vi "TEST-SERIALIZE.vi"() -> ()   [LabVIEW 2019]
uses:
  Response--Variant--Cluster.ctl
  Response--String--Cluster.ctl
  83b9611c-e125-4a79-a28c-7d3b3a1c2440.vi
  eb13c5f8-5704-4e01-b19a-e5499a693321.vi
  35bd3d0d-1b36-4666-bfef-67306258898e.vi
  db572bd4-01e3-4c34-87d8-1273e3f61b28.vi
  9ae522ea-7a25-4ffe-8949-55076a4dedc3.vi
  1886c53c-c316-4cc4-aec7-e01830886c52.vi
  2ae47432-6b04-43af-b607-7b3945031cca.vi
  7945c8ed-bd74-4a6a-aaee-7dd52200f6b1.vi
  83b9611c-e125-4a79-a28c-7d3b3a1c2440.vi/16d22996-583c-4114-be7f-826d89ca4985.vi
  9ae522ea-7a25-4ffe-8949-55076a4dedc3.vi/34417eb6-c264-4261-ab76-2576b9b9ebac.vi
  lv-venv/lv.lib/vi.lib/JDP Science/JSONtext/Variant to JSON Text.vi
  <vilib>/Utility/sysdir.llb/Get System Directory.vi
  lv-venv/lv.lib/vi.lib/JDP Science/JSONtext/JSON text to Variant.vi
  lv-venv/lv.lib/vi.lib/JDP Science/JSONtext/LVClass Serializer/JSONtext LVClass Serializer.lvclass
  lv-venv/lv.lib/vi.lib/addons/_JKI.lib/Serialization/JSON/JKI JSON Serialization.lvlib
panel:
  out "serialize":dbl
  out "Numeric":i32
  out "spreadsheet string":string
  out "XY Graph":cluster{i32[], dbl[]}[](graph)
  out "Array":i32[](array[numeric])
  out "data":i32[](array[numeric])
  out "serialize JSON":dbl[](array[numeric]) format="%#_6p"
  out "{JSON}":string
  out "id":string
  out "parse JSON":dbl[](array[numeric]) format="%#_6p"
  in  "Enum":T1(ring)
  out "x = y?":bool
  in  "Max Array Size":i32=100 format="%.0p"
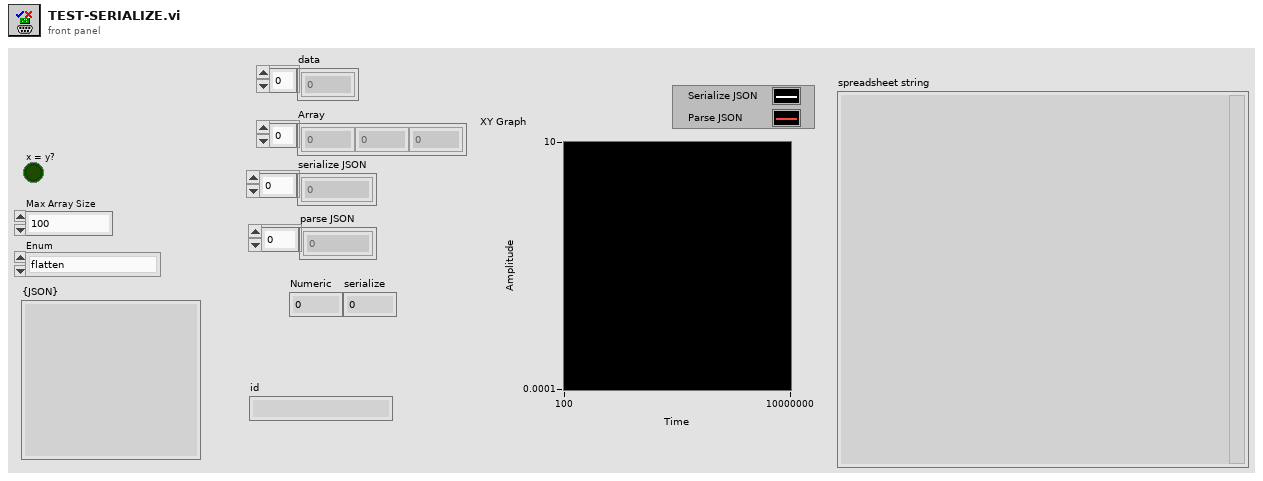
[diagram p1: front panel]
types:
  T1 = enum16{"flatten", "JKI JSON", "JKI JSON + flatten", "JSONtext", "JSONtext + flatten", "myJSON + flatten", "PythonModule"}
  T2 = typedef "Response--Variant--Cluster.ctl" = cluster{"jsonrpc":string, "result":variant, "id":string}
  T3 = typedef "Response--String--Cluster.ctl" = cluster{"jsonrpc":string, "result":string, "id":string}
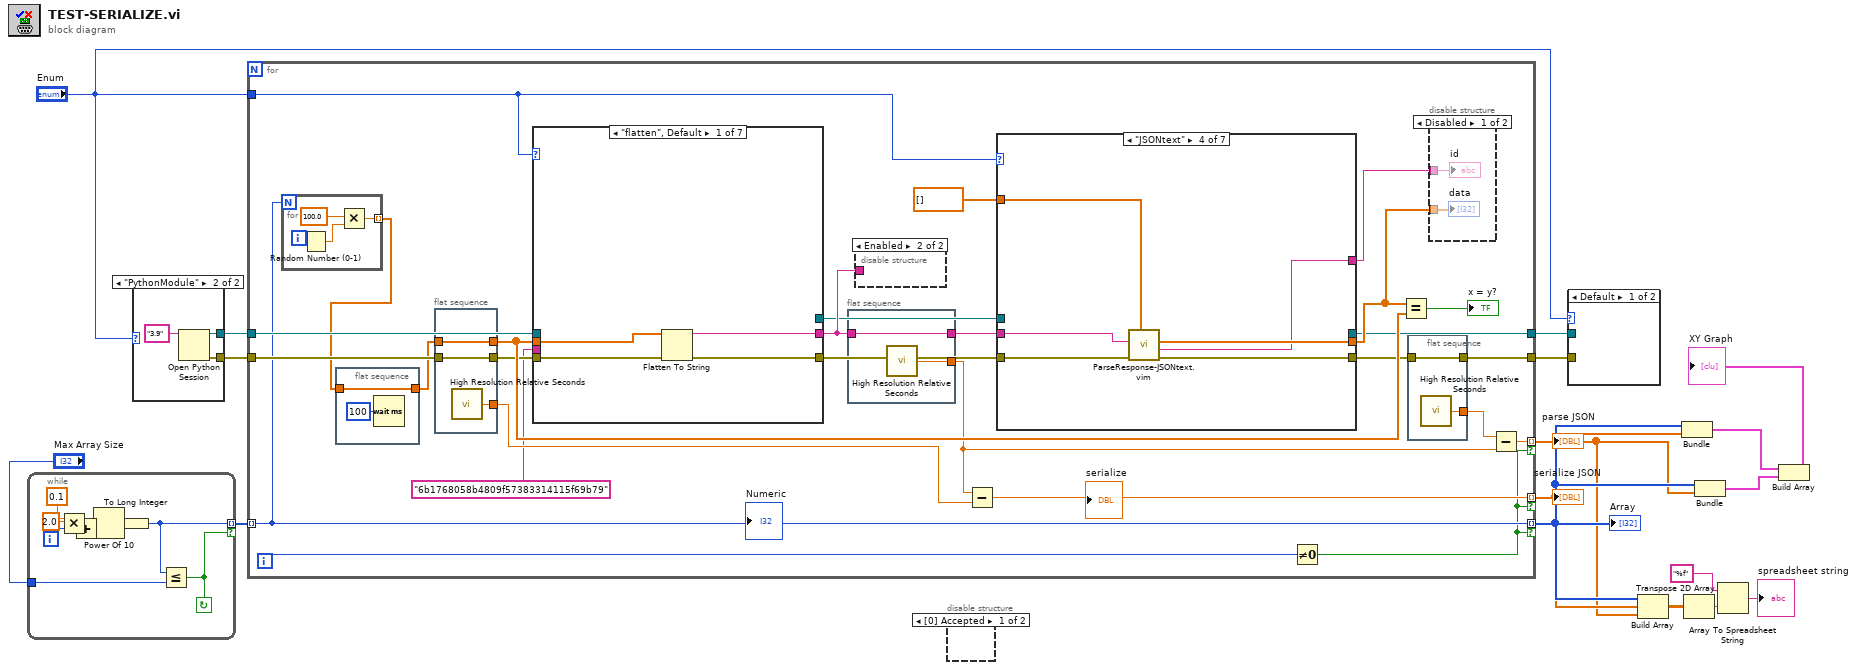
[diagram p0: block diagram]
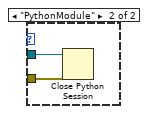
[diagram p3: hidden frame]
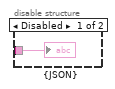
[diagram p5: hidden frame]
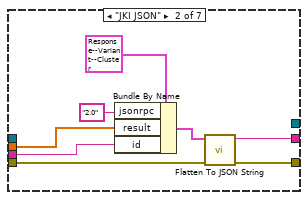
[diagram p6: hidden frame]
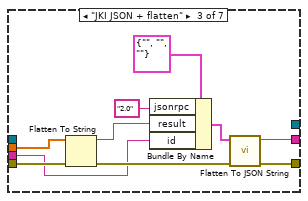
[diagram p7: hidden frame]
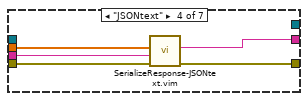
[diagram p8: hidden frame]
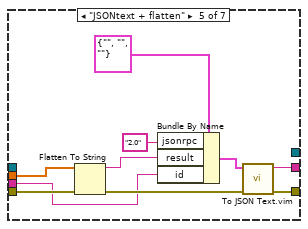
[diagram p9: hidden frame]
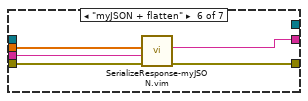
[diagram p10: hidden frame]
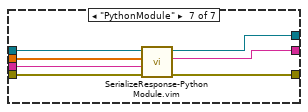
[diagram p11: hidden frame]
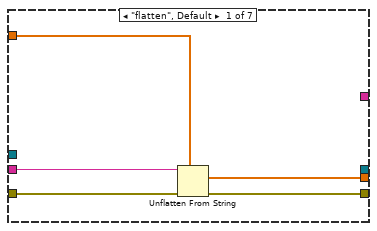
[diagram p12: hidden frame]
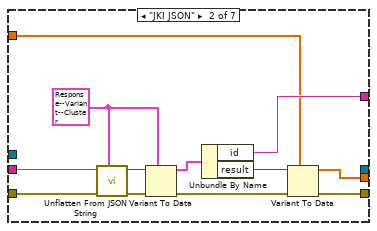
[diagram p13: hidden frame]
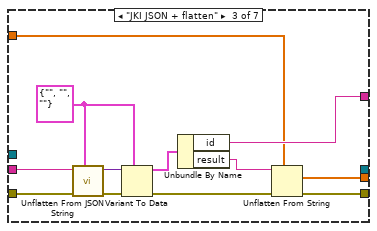
[diagram p14: hidden frame]
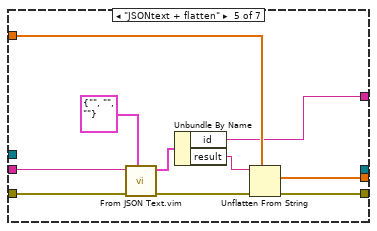
[diagram p15: hidden frame]
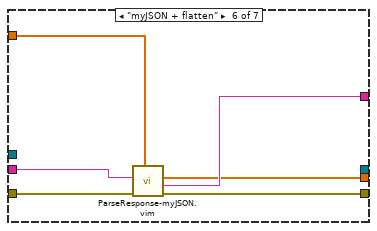
[diagram p16: hidden frame]
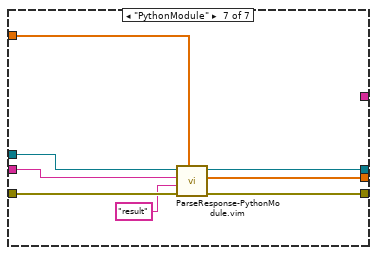
[diagram p17: hidden frame]
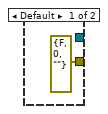
[diagram p18: hidden frame]
diagram:
  n1 = while {
    tunnel: [w18] -> w14 mode=indexing if=w23
    tunnel: "Max Array Size" -> [w22]
    i -> [w26]
    stop <- w23 continue-if-true
    n2 = Multiply(x=0.1, y=w26) -> (x*y=w24:dbl)
    n3 = Add(x=w24, y=2.0) -> (x+y=w20:dbl)
    n4 = Power Of 10(x=w20) -> (10^x=w21:dbl)
    n5 = To Long Integer(number=w21) -> (32bit integer=w18:i32)
    n6 = Less Or Equal?(x=w18, y=w22) -> (x <= y?=w23:bool)
  }
  n7 = case shown="\"PythonModule\"" "Enum" {
    tunnel: [errorcluster {"status"=FALSE, "code"=0, "source"=""} ("error in (no error)") w29] -> w17
    tunnel: [_ w28] -> w16
    frame Default {
    }
    frame "PythonModule" {
      n8 = Open Python Session(python version="3.9" ("Python version")) -> (session out=w28:refnum<k35>, error out=w29:errorcluster)  [unwired: 2 in]
    }
  }
  n9 = for {
    tunnel: [w49] -> w6 mode=indexing if=w35
    tunnel: [w45] -> w5 mode=indexing if=w35
    tunnel: w17 -> [w42]
    tunnel: w16 -> [w41]
    tunnel: "Enum" -> [w40]
    tunnel: w14 -> [w37] mode=indexing
    tunnel: [w37] -> w7 mode=indexing if=w35
    tunnel: [w34] -> w10
    tunnel: [w33] -> w9
    i -> [w36]
    n10 = for {
      N: w37 -> [_]
      tunnel: [w179] -> w31 mode=indexing
      n11 = Random Number (0-1)() -> (number: 0 to 1=w178:dbl)
      n12 = Multiply(x=100.0, y=w178) -> (x*y=w179:dbl)
    }
    n13 = flat-sequence {
      tunnel: w31 -> [w59]
      tunnel: [w59] -> w32
      frame #0 {
        n14 = Wait (ms)(milliseconds to wait=u32 100) -> ()  [unwired: 1 out]
      }
    }
    n15 = flat-sequence {
      tunnel: [w68] -> w56
      tunnel: [w69] -> w51
      tunnel: w32 -> [w68]
      tunnel: [w67] -> w48
      tunnel: w42 -> [w67]
      frame #0 {
        n16 = call <vilib>:"High Resolution Relative Seconds.vi"() -> ("relative seconds"=w69:dbl)
      }
    }
    n17 = case shown="\"flatten\", Default" w40 {
      tunnel: w56 -> [w73 w79 w91 w93 w104 w108 w118]
      tunnel: [w70 w76 w85 w96 w100 w111 w115] -> w46
      tunnel: w48 -> [w71 w77 w87 w95 w102 w110 w112]
      tunnel: "6b1768058b4809f57383314115f69b79" -> [_ w74 w82 w94 w97 w109 w117]
      tunnel: [w72 w78 w88 w92 w103 w107 w116] -> w44
      tunnel: [_ _ _ _ _ _ w114] -> w43
      tunnel: w41 -> [_ _ _ _ _ _ w113]
      frame "flatten", Default {
        n18 = Flatten To String(anything=w73, error in (no error)=w71) -> (data string=w72:string, error out=w70:errorcluster)  [unwired: 2 in, 1 out]
      }
      frame "JKI JSON" {
        n19 = Bundle By Name(cluster=T2 {"jsonrpc"="", "result"=variant, "id"=""} ("response"), "jsonrpc"="2.0", "result"=w79, "id"=w74) -> (w80:T2)
        n20 = call "Flatten To JSON String.vi"("error in (no error)"=w77, "Variant"=w80) -> ("error out"=w76:errorcluster, "JSON String"=w78:string)  [unwired: 8 in]
      }
      frame "JKI JSON + flatten" {
        n21 = Flatten To String(anything=w91, error in (no error)=w87) -> (data string=w84:string, error out=w86:errorcluster)  [unwired: 2 in, 1 out]
        n22 = Bundle By Name(cluster=T3 {"jsonrpc"="", "result"="", "id"=""} ("response"), "jsonrpc"="2.0", "result"=w84, "id"=w82) -> (w83:T3)
        n23 = call "Flatten To JSON String.vi"("error in (no error)"=w86, "Variant"=w83) -> ("error out"=w85:errorcluster, "JSON String"=w88:string)  [unwired: 8 in]
      }
      frame "JSONtext" {
        n24 = call "SerializeResponse-JSONtext.vim"("error in (no error)"=w95, "id"=w94, "result"=w93) -> ("error out"=w96:errorcluster, "<JSON>"=w92:string)  [unwired: 7 in]
      }
      frame "JSONtext + flatten" {
        n25 = Flatten To String(anything=w104, error in (no error)=w102) -> (data string=w101:string, error out=w99:errorcluster)  [unwired: 2 in, 1 out]
        n26 = Bundle By Name(cluster=T3 {"jsonrpc"="", "result"="", "id"=""} ("response 2"), "jsonrpc"="2.0", "result"=w101, "id"=w97) -> (w105:T3)
        n27 = call "To JSON Text.vim"("error in (no error)"=w99, "Anything"=w105) -> ("error out"=w100:errorcluster, "<JSON>"=w103:string)  [unwired: 8 in]
      }
      frame "myJSON + flatten" {
        n28 = call "SerializeResponse-myJSON.vim"("error in (no error)"=w110, "id"=w109, "result"=w108) -> ("error out"=w111:errorcluster, "{JSON}"=w107:string)  [unwired: 7 in]
      }
      frame "PythonModule" {
        n29 = call "SerializeResponse-PythonModule.vim"("error in (no error)"=w112, "id"=w117, "Response"=w118, "session in"=w113) -> ("error out"=w115:errorcluster, "{JSON}"=w116:string, "session out"=w114:refnum<k35>)  [unwired: 5 in]
      }
    }
    n30 = flat-sequence {
      tunnel: w44 -> [w64]
      tunnel: [w64] -> w52
      tunnel: [w63] -> w50
      frame #0 {
        n31 = call <vilib>:"High Resolution Relative Seconds.vi"() -> ("relative seconds"=w63:dbl)
      }
    }
    n32 = disable-structure shown="Enabled" {
      disable-tunnel: w44 -> [w62 _]
      frame Disabled {
        "{JSON}" <- w62
      }
      frame Enabled {
      }
    }
    n33 = Subtract(x=w50, y=w51) -> (x-y=w49:dbl)
    "serialize" <- w49
    n34 = case shown="\"JSONtext\"" w40 {
      tunnel: [w123 w135 w147 w152 w162 w169 w170] -> w53
      tunnel: [w119 w134 w146 w151 w154 w164 w172] -> w54
      tunnel: dbl[] [] ("data") -> [w120 w124 w136 w150 w158 w167 w173]
      tunnel: [_ w125 w137 w148 w155 w165 _] -> w38
      tunnel: w52 -> [w122 w128 w140 w149 w160 w166 w174]
      tunnel: w46 -> [w121 w127 w138 w153 w159 w168 w176]
      tunnel: w43 -> [_ _ _ _ _ _ w177]
      tunnel: [_ _ _ _ _ _ w171] -> w33
      frame "flatten", Default {
        n35 = Unflatten From String(type=w120, binary string=w122, error in (no error)=w121) -> (value=w119:dbl[], error out=w123:errorcluster)  [unwired: 2 in, 1 out]
      }
      frame "JKI JSON" {
        w126 = T2 {"jsonrpc"="", "result"=variant, "id"=""} ("response")
        n36 = call "Unflatten From JSON String.vi"("Type and Defaults"=w126, "error in (no error)"=w127, "JSON String"=w128) -> ("error out"=w131:errorcluster, "Variant"=w133:variant)  [unwired: 7 in]
        n37 = Variant To Data(error in=w131, type=w126, Variant=w133) -> (data=w132:T2, error out=w129:errorcluster)
        n38 = Unbundle By Name(w132) -> ("id"=w125:string, "result"=w130:variant)
        n39 = Variant To Data(error in=w129, type=w124, Variant=w130) -> (data=w134:dbl[], error out=w135:errorcluster)
      }
      frame "JKI JSON + flatten" {
        w139 = T3 {"jsonrpc"="", "result"="", "id"=""} ("response")
        n40 = call "Unflatten From JSON String.vi"("Type and Defaults"=w139, "error in (no error)"=w138, "JSON String"=w140) -> ("error out"=w143:errorcluster, "Variant"=w145:variant)  [unwired: 7 in]
        n41 = Variant To Data(error in=w143, type=w139, Variant=w145) -> (data=w144:T3, error out=w141:errorcluster)
        n42 = Unbundle By Name(w144) -> ("id"=w137:string, "result"=w142:string)
        n43 = Unflatten From String(type=w136, binary string=w142, error in (no error)=w141) -> (value=w146:dbl[], error out=w147:errorcluster)  [unwired: 2 in, 1 out]
      }
      frame "JSONtext" {
        n44 = call "ParseResponse-JSONtext.vim"("result"=w150, "error in (no error)"=w153, "{JSON}"=w149) -> ("error out"=w152:errorcluster, "id"=w148:string, "result"=w151:dbl[])  [unwired: 6 in]
      }
      frame "JSONtext + flatten" {
        n45 = call "From JSON Text.vim"("Data Type and Default Value"=T3 {"jsonrpc"="", "result"="", "id"=""} ("response 2"), "error in (no error)"=w159, "JSON"=w160) -> ("error out"=w156:errorcluster, "Data out"=w163:T3)  [unwired: 7 in]
        n46 = Unbundle By Name(w163) -> ("id"=w155:string, "result"=w161:string)
        n47 = Unflatten From String(type=w158, binary string=w161, error in (no error)=w156) -> (value=w154:dbl[], error out=w162:errorcluster)  [unwired: 2 in, 1 out]
      }
      frame "myJSON + flatten" {
        n48 = call "ParseResponse-myJSON.vim"("datatype"=w167, "error in (no error)"=w168, "{JSON}"=w166) -> ("error out"=w169:errorcluster, "id"=w165:string, "data out"=w164:dbl[])  [unwired: 5 in, 1 out]
      }
      frame "PythonModule" {
        n49 = call "ParseResponse-PythonModule.vim"("Response Type"=w173, "error in (no error)"=w176, "Key"="result", "{JSON}"=w174, "session in"=w177) -> ("error out"=w170:errorcluster, "Response"=w172:dbl[], "session out"=w171:refnum<k35>)  [unwired: 4 in]
      }
    }
    n50 = Not Equal To 0?(x=w36) -> (x != 0?=w35:bool)
    n51 = Equal?(x=w54, y=w56) -> (x = y?=→"x = y?":bool)
    n52 = flat-sequence {
      tunnel: [w66] -> w57
      tunnel: w53 -> [w65]
      tunnel: [w65] -> w34
      frame #0 {
        n53 = call <vilib>:"High Resolution Relative Seconds.vi"() -> ("relative seconds"=w66:dbl)
      }
    }
    n54 = disable-structure shown="Disabled" {
      disable-tunnel: w54 -> [w61 _]
      disable-tunnel: w38 -> [w60 _]
      frame Disabled {
        "data" <- w61
        "id" <- w60
      }
      frame Enabled {
      }
    }
    n55 = Subtract(x=w57, y=w50) -> (x-y=w45:dbl)
    "Numeric" <- w37
  }
  "parse JSON" <- w5
  "serialize JSON" <- w6
  "Array" <- w7
  n56 = disable-structure shown="[0] Accepted" {
    frame Enabled {
    }
    frame Disabled {
    }
  }
  n57 = case shown="Default" "Enum" {
    tunnel: w10 -> [_ w182]
    tunnel: w9 -> [_ w181]
    frame Default {
    }
    frame "PythonModule" {
      n58 = Close Python Session(session in=w181, error in=w182) -> ()  [unwired: 1 out]
    }
  }
  n59 = Build Array(w7, w6, w5) -> (w4:dbl[][])
  n60 = Bundle(w7, w6) -> (w13:cluster{i32[], dbl[]})  [unwired: 1 in]
  n61 = Transpose 2D Array(2D array=w4) -> (transposed array=w1:dbl[][])
  n62 = Bundle(w7, w5) -> (w12:cluster{i32[], dbl[]})  [unwired: 1 in]
  n63 = Array To Spreadsheet String(array=w1, 3:"%f" ("format string")) -> (spreadsheet string=→"spreadsheet string":string)  [unwired: 1 in]
  n64 = Build Array(w13, w12) -> (→"XY Graph":cluster{i32[], dbl[]}[])
